vi "destroy Renderer.vi"(11 "pRendererId":i32) -> (3 "function return":i32)   [LabVIEW 2012, in "cvlib.lvlib"]
doc: "extern \"C\" __declspec(dllexport) long __cdecl destroyRenderer( long pRendererId);"
uses:
  cvlib.lvlib
  cvlib.dll
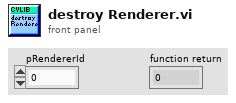
[diagram p1: front panel]
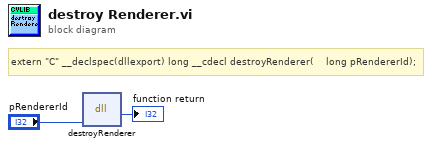
[diagram p0: block diagram]
diagram:
  # "extern \"C\" __declspec(dllexport) long __cdecl destroyRenderer(\t\t\t\tlong pRendererId);"
  n1 = dll-call lib="C:/Users/myerslab/workspace2/Libraries/ClearVolume/cpp/labview/lvcvlib/cvlib.*" fn="destroyRenderer"("pRendererId"="pRendererId") -> (→"function return":i32)  [unwired: 4 in, 2 out]
